vi "Werkseinstellung erstellen.vi"(8 "error in (no error)":errorcluster caption="Fehler (Eingang, kein Fehler)") -> (0 "error out":errorcluster caption="Fehler (Ausgang)")   [LabVIEW 2020, in "allgemeine Sub-VIs.lvlib"]
uses:
  allgemeine Sub-VIs.lvlib
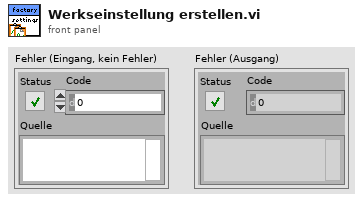
[diagram p1: front panel]
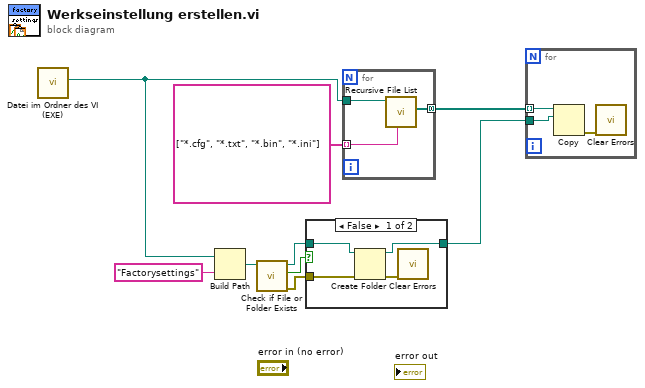
[diagram p0: block diagram]
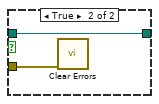
[diagram p2: hidden frame]
diagram:
  n1 = call "Datei im Ordner des VI (EXE).vi"() -> ("Ordner des Haupt-VIs"=w3:path)  [unwired: 9 in, 2 out]
  n2 = Build Path(base path=w3, name or relative path="Factorysettings" ("Name oder relativer Pfad")) -> (appended path=w4:path)
  n3 = call <vilib>:"Check if File or Folder Exists.vi"("path"=w4) -> ("error out"=w8:errorcluster, "file or folder exists?"=w7:bool, "dup path"=w9:path)  [unwired: 8 in]
  n4 = case shown="False" w7 {
    tunnel: w9 -> [w13 w15]
    tunnel: w8 -> [w12 w14]
    tunnel: [w11 w15] -> w5
    frame False {
      n5 = Create Folder(path (use dialog)=w13, error in=w12) -> (created path=w11:path, error out=w10:errorcluster)  [unwired: 1 in, 1 out]
      n6 = call <vilib>:"Clear Errors.vi"("error in (no error)"=w10) -> ()  [unwired: 5 in, 2 out]
    }
    frame True {
      n7 = call <vilib>:"Clear Errors.vi"("error in (no error)"=w14) -> ()  [unwired: 5 in, 2 out]
    }
  }
  n8 = for {
    tunnel: string[] ["*.cfg", "*.txt", "*.bin", "*.ini"] ("Dateinamen") -> [w18] mode=indexing
    tunnel: w3 -> [w17]
    tunnel: [w16] -> w1 mode=concatenating
    n9 = call <vilib>:"Recursive File List.vi"("pattern"=w18, "Folder Path"=w17) -> ("All Files in Dir"=w16:path[])  [unwired: 5 in, 4 out]
  }
  n10 = for {
    tunnel: w5 -> [w21]
    tunnel: w1 -> [w19] mode=indexing
    n11 = Copy(10:w21, 11:w19) -> (0:w20:errorcluster)  [unwired: 3 in, 2 out]
    n12 = call <vilib>:"Clear Errors.vi"("error in (no error)"=w20) -> ()  [unwired: 5 in, 2 out]
  }
